vi "parser_01.vi"(4 "data in":string) -> (1 "Exit":bool, 2 "Answer":string)   [LabVIEW 2010]
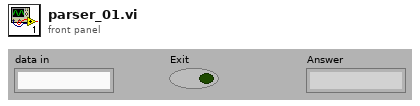
[diagram p1: front panel]
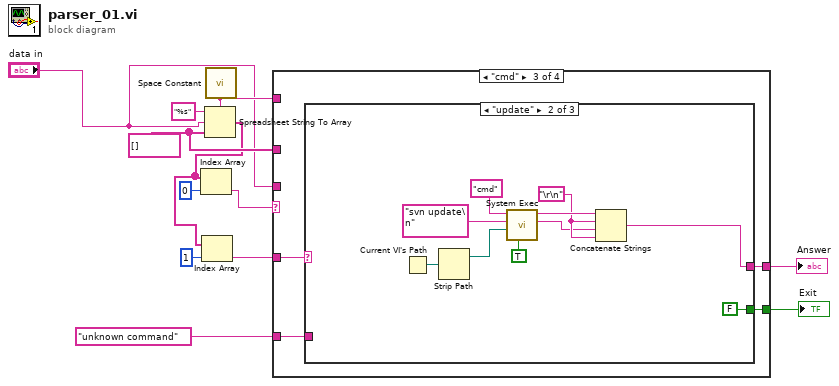
[diagram p0: block diagram]
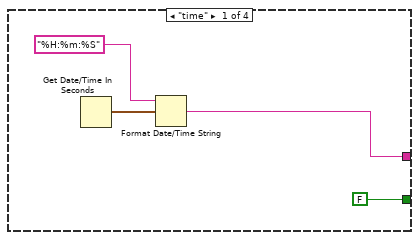
[diagram p2: hidden frame]
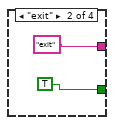
[diagram p3: hidden frame]
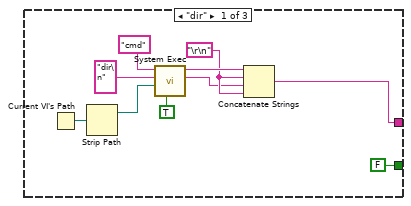
[diagram p4: hidden frame]
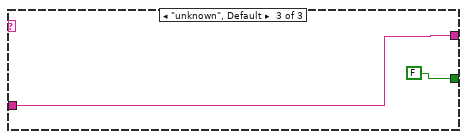
[diagram p5: hidden frame]
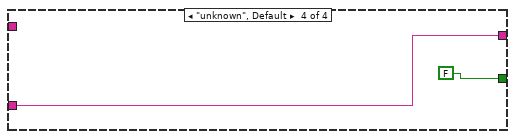
[diagram p6: hidden frame]
diagram:
  w7 = string[] []
  n1 = call <vilib>:"Space Constant.vi"() -> ("String"=w6:string)
  n2 = Spreadsheet String To Array(delimiter (Tab)=w6, format string="%s", spreadsheet string="data in", array type (2D Dbl)=w7) -> (array=w3:string[])
  n3 = Index Array(array=w3, index=0) -> (element=w10:string)
  n4 = Index Array(array=w3, index=1) -> (element=w2:string)
  n5 = case shown="\"cmd\"" w10 {
    tunnel: [w14 "exit" w22 w45] -> w8
    tunnel: [FALSE TRUE w21 FALSE] -> w9
    tunnel: w7 -> [_ _ _ _]
    tunnel: w6 -> [_ _ _ _]
    tunnel: "data in" -> [_ _ _ _]
    tunnel: w2 -> [_ _ w20 _]
    tunnel: "unknown command" -> [_ _ w19 w45]
    frame "time" {
      n6 = Get Date/Time In Seconds() -> (seconds since 1Jan1904=w16:timestamp)
      n7 = Format Date/Time String(time format string (%c)="%H:%m:%S", seconds (now)=w16) -> (date/time string=w14:string)  [unwired: 1 in]
    }
    frame "exit" {
    }
    frame "cmd" {
      n8 = case shown="\"update\"" w20 {
        tunnel: [w24 w34 w43] -> w22
        tunnel: [FALSE FALSE FALSE] -> w21
        tunnel: w19 -> [_ _ w43]
        frame "dir" {
          w28 = "\r\n"
          n9 = Current VI's Path() -> (path=w30:path)
          n10 = Strip Path(path=w30) -> (stripped path=w31:path)  [unwired: 1 out]
          n11 = call <vilib>:"System Exec.vi"("run minimized? (F)"=TRUE, "working directory"=w31, "standard input"="dir\n" ("command line"), "command line"="cmd") -> ("standard error"=w27:string, "standard output"=w32:string)  [unwired: 4 in, 2 out]
          n12 = Concatenate Strings(w32, w28, w27, w28) -> (w24:string)
        }
        frame "update" {
          w38 = "\r\n"
          n13 = Current VI's Path() -> (path=w40:path)
          n14 = Strip Path(path=w40) -> (stripped path=w41:path)  [unwired: 1 out]
          n15 = call <vilib>:"System Exec.vi"("run minimized? (F)"=TRUE, "working directory"=w41, "standard input"="svn update\n" ("command line"), "command line"="cmd") -> ("standard error"=w37:string, "standard output"=w42:string)  [unwired: 4 in, 2 out]
          n16 = Concatenate Strings(w42, w38, w37, w38) -> (w34:string)
        }
        frame "unknown", Default {
        }
      }
    }
    frame "unknown", Default {
    }
  }
  "Exit" <- w9
  "Answer" <- w8
